vi "HAL camera stop.vi"   [LabVIEW 2016]
uses:
  Camera/camera globals.vi
  Atmcd32d.dll
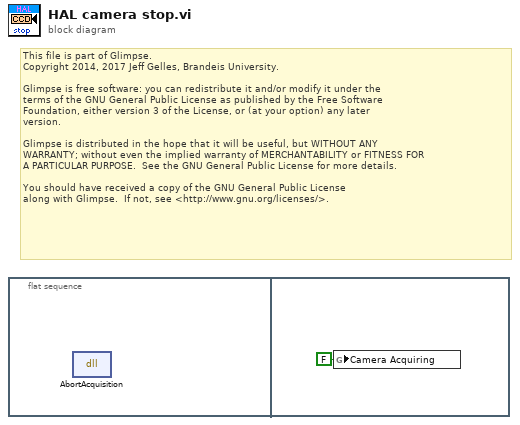
[diagram p0: block diagram]
diagram:
  # "This file is part of Glimpse. \nCopyright 2014, 2017 Jeff Gelles, Brandeis University.    \n\nGlimpse is free software: you can redistribute it and/or modify it under the \nterms of the GNU General Public License as published by the Free Software \nFoundation, either version 3 of the License, or (at your option) any later \nversion.\n\nGlimpse is distributed in the hope that it will be useful, but WITHOUT ANY \nWARRANTY; without even the implied warranty of MERCHANTABILITY or FITNESS FOR \nA PARTICULAR PURPOSE.  See the GNU General Public License for more details.\n\nYou should have received a copy of the GNU General Public License\nalong with Glimpse.  If not, see <http://www.gnu.org/licenses/>."
  n1 = flat-sequence {
    frame #0 {
      n2 = dll-call lib="ATMCD32D.DLL" fn="AbortAcquisition" label="Call Library Function\nAbort"() -> ()  [unwired: 3 in, 3 out]
    }
    frame #1 {
      n3 = global write "camera globals.vi" "Camera Acquiring"(FALSE ("Andor Aquiring")) -> ()
    }
  }
